vi "Pre Launch Init.vi"(11 "startconteo in":refnum<class "startconteo.lvclass">) -> (0 "error out":errorcluster, 3 "startconteo out":refnum<class "startconteo.lvclass">)   [LabVIEW 2019, in "startconteo.lvlib" / "startconteo.lvclass"]
doc: "(<B>Filename</B>: Actor Framework.lvlib:Actor.lvclass:Pre Launch Init.vi)\n\nDefines behavior that occurs after the Launch Nested Actor method is invoked but before the actor's Actor Core method begins running.\n\nBy default, this method does nothing. A descendant class may override it to define behavior."
uses:
  startconteo.lvclass
  startconteo.lvclass/startconteo.ctl
  <vilib>/ActorFramework/Actor/Actor.lvclass
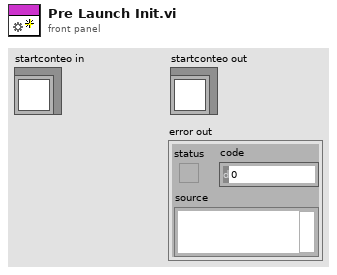
[diagram p1: front panel]
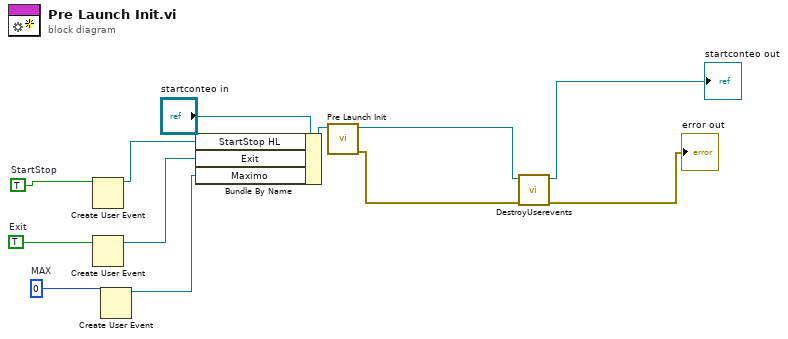
[diagram p0: block diagram]
diagram:
  w2 = 0  # MAX
  w4 = TRUE  # Exit
  w11 = TRUE  # StartStop
  n1 = Create User Event(user event datatype=w11) -> (user event=w9:refnum<user-event>)  [unwired: 1 in, 1 out]
  n2 = Create User Event(user event datatype=w4) -> (user event=w3:refnum<user-event>)  [unwired: 1 in, 1 out]
  n3 = Create User Event(user event datatype=w2) -> (user event=w1:refnum<user-event>)  [unwired: 1 in, 1 out]
  n4 = Bundle By Name(cluster="startconteo in", "StartStop HL"=w9, "Exit"=w3, "Maximo"=w1) -> (w10:refnum<class "startconteo.lvclass">)
  n5 = call-parent "Pre Launch Init.vi"("Actor in"=w10) -> ("error out"=w8:errorcluster, "Actor out"=w6:refnum<class "startconteo.lvclass">)  [unwired: 9 in]
  n6 = call "DestroyUserevents.vi"("error in (no error)"=w8, "startconteo in"=w6) -> ("error out"=→"error out":errorcluster, "startconteo out"=→"startconteo out":refnum<class "startconteo.lvclass">)  [unwired: 8 in]
